vi "test_over.vi"() -> ()   [LabVIEW 2013]
uses:
  <vilib>/Utility/file.llb/Write To Spreadsheet File (string).vi
panel:
  out "subarray 2":string[][](array[string])
  out "subarray":string[][](array[string])
  out "size(s)":i32
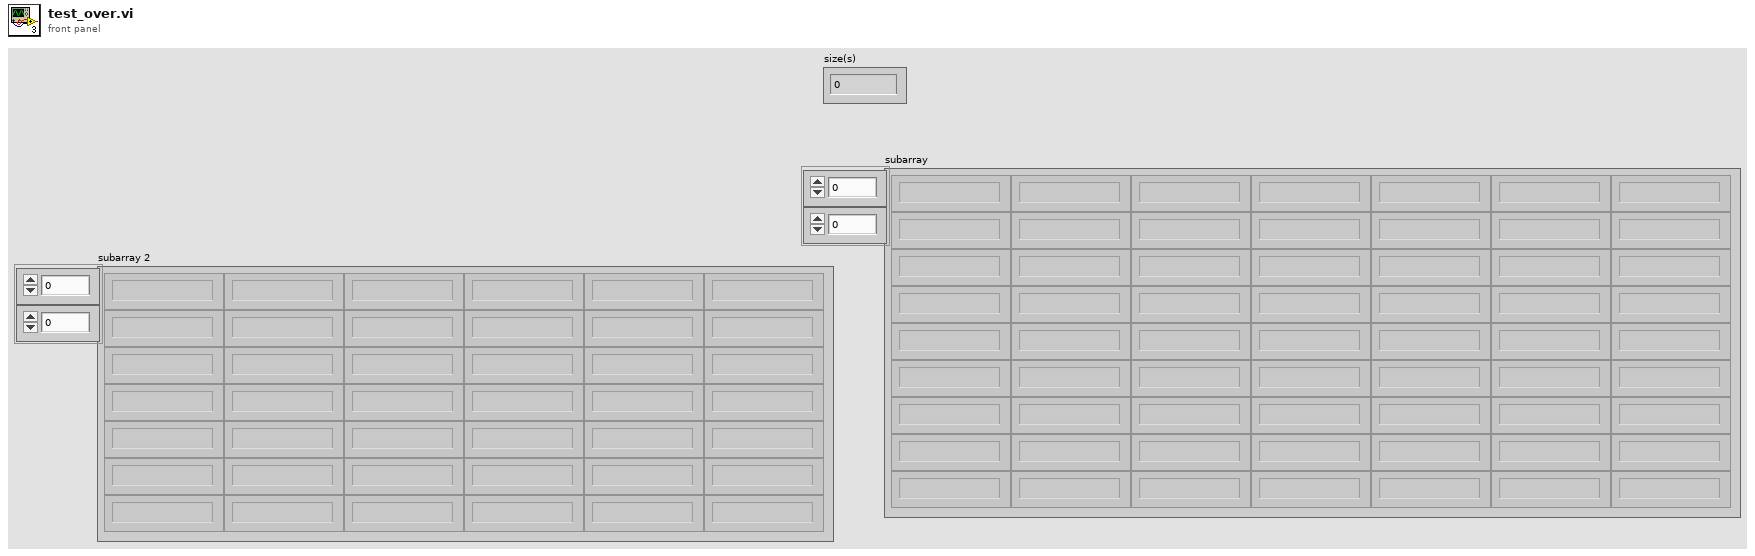
[diagram p1: front panel]
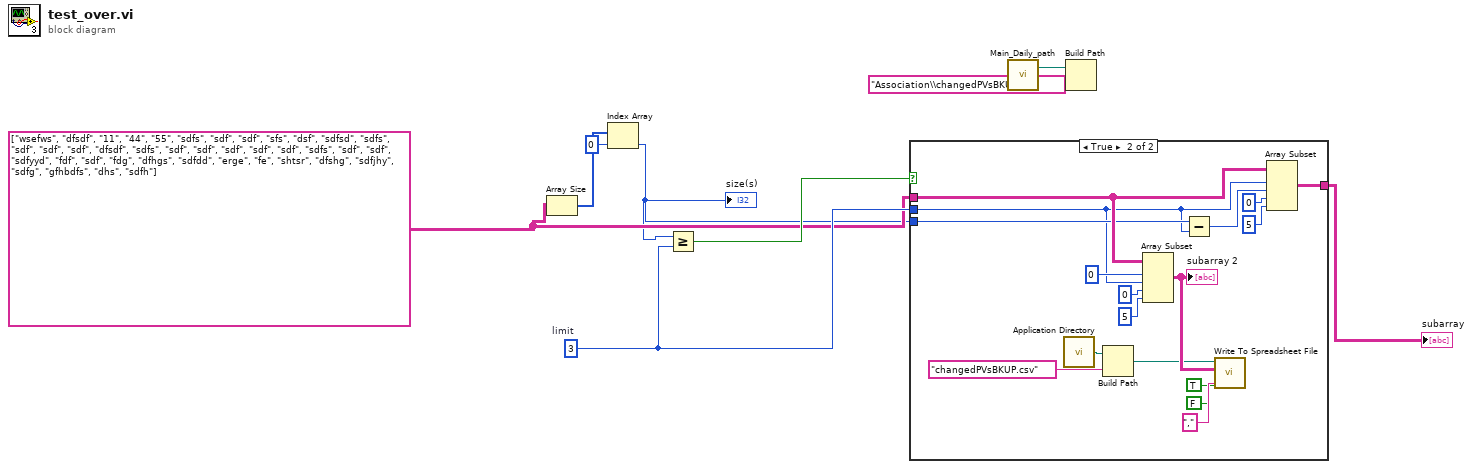
[diagram p0: block diagram]
diagram:
  w8 = 3  # limit
  w6 = string[][] [["wsefws", "dfsdf", "11", "44", "55"], ["sdfs", "sdf", "sdf", "sfs", "dsf"], ["sdfsd", "sdfs", "sdf", "sdf", "sdf"], ["dfsdf", "sdfs", "sdf", "sdf", "sdf"], ["sdf", "sdf", "sdfs", "sdf", "sdf"], ["sdfyyd", "fdf", "sdf", "fdg", "dfhgs"], ["sdfdd", "erge", "fe", "shtsr", "dfshg"], ["sdfjhy", "sdfg", "gfhbdfs", "dhs", "sdfh"]] ("Diff list")
  n1 = Array Size(array=w6) -> (size(s)=w5:i32[])
  n2 = Index Array(array=w5, index=0) -> (element=w3:i32)
  "size(s)" <- w3
  n3 = Greater Or Equal?(x=w3, y=w8) -> (x >= y?=w7:bool)
  n4 = case shown="True" w7 {
    tunnel: w6 -> [w10 w21]
    tunnel: [w10 w25] -> w9
    tunnel: w3 -> [_ w13]
    tunnel: w8 -> [_ w12]
    frame False {
    }
    frame True {
      n5 = call <vilib>:"Application Directory.vi"() -> ("Application Directory"=w19:path)
      n6 = Build Path(base path=w19, name or relative path="changedPVsBKUP.csv") -> (appended path=w17:path)
      n7 = Array Subset(array=w21, index (row)=0 ("index"), length (row)=w12, index (col)=0 ("index"), length (col)=5 ("length")) -> (w20:string[][])
      "subarray 2" <- w20
      n8 = Subtract(x=w13, y=w12) -> (x-y=w11:i32)
      n9 = call-poly <vilib>:"Write To Spreadsheet File.vi"("delimiter (\\t)"="," ("delimiter (\\t)"), "transpose? (no:F)"=FALSE, "append to file? (new file:F)"=TRUE, "2D data"=w20, "file path (dialog if empty)"=w17) -> ()  [unwired: 3 in, 1 out]
      n10 = Array Subset(array=w21, index (row)=w12, length (row)=w11, index (col)=0 ("index"), length (col)=5 ("length")) -> (w25:string[][])
    }
  }
  "subarray" <- w9
  n11 = call "Main_Daily_path.vi"() -> ("Directory path"=w2:path)  [unwired: 10 in, 1 out]
  n12 = Build Path(base path=w2, name or relative path="Association\\changedPVsBKUP.csv" ("string")) -> ()  [unwired: 1 out]
